vi "MattFileCreator-v9.vi"(6 "Comments":T5, 8 "Input Array":dbl[](array[numeric]), 9 "File path":path, 10 "table":string, 11 "connection reference":T6) -> (0 "error out":errorcluster, 3 "connection reference out":T6)   [LabVIEW 2014]
uses:
  <vilib>/addons/database/Connection.llb/Conn ObjectReference.ctl
  <vilib>/addons/database/NI_Database_API.lvlib
panel:
  out "output cluster 4":T1
  out "output cluster 3":T2
  out "output cluster 2":T3
  out "output cluster":T4
  in  "Database input":T7
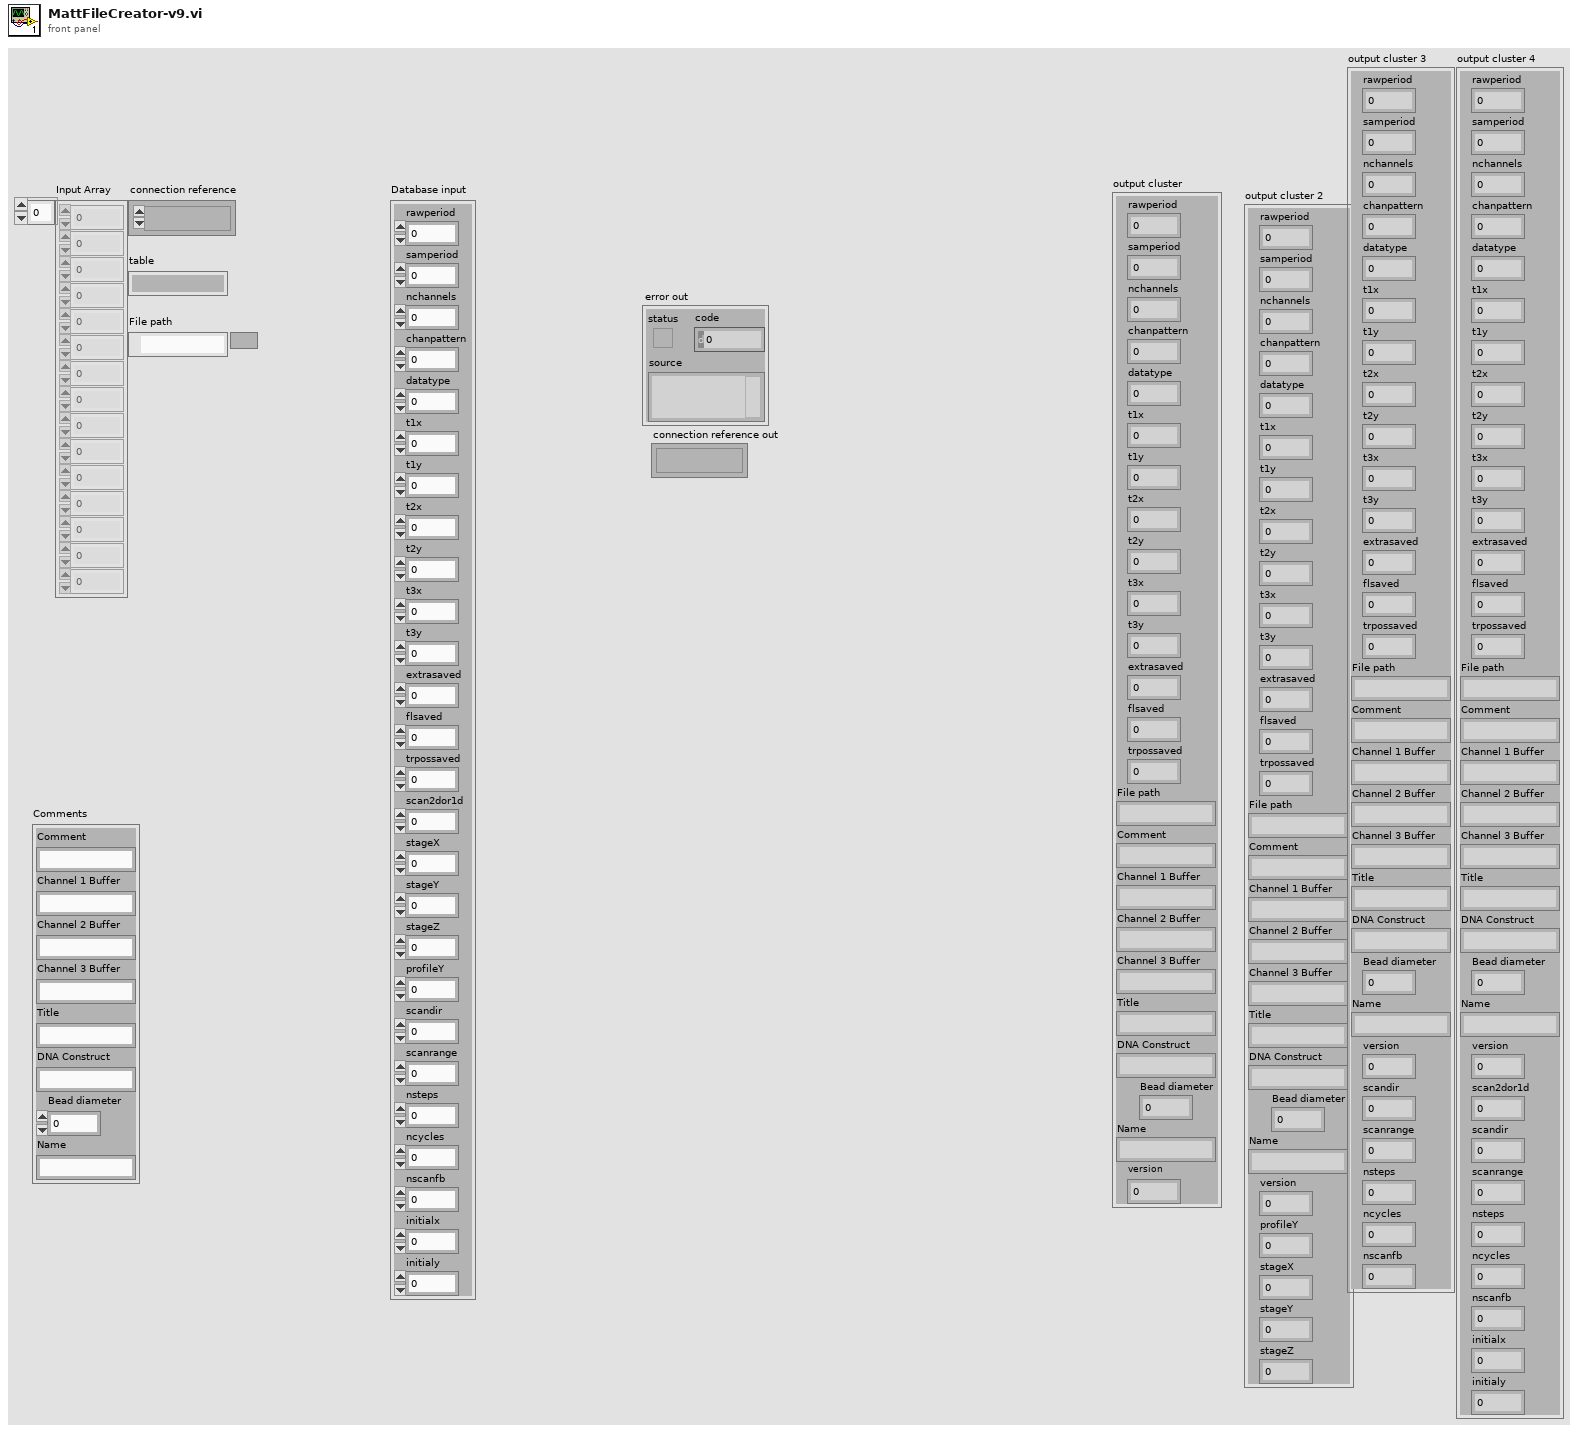
[diagram p1: front panel]
types:
  T1 = cluster{"rawperiod":dbl, "samperiod":dbl, "nchannels":dbl, "chanpattern":dbl, "datatype":dbl, "t1x":dbl, "t1y":dbl, "t2x":dbl, "t2y":dbl, "t3x":dbl, "t3y":dbl, "extrasaved":dbl, "flsaved":dbl, "trpossaved":dbl, "File path":string, "Comment":string, "Channel 1 Buffer":string, "Channel 2 Buffer":string, "Channel 3 Buffer":string, "Title":string, "DNA Construct":string, "Bead diameter":dbl, "Name":string, "version":i32, "scan2dor1d":dbl, "scandir":dbl, "scanrange":dbl, "nsteps":dbl, "ncycles":dbl, "nscanfb":dbl, "initialx":dbl, "initialy":dbl}
  T2 = cluster{"rawperiod":dbl, "samperiod":dbl, "nchannels":dbl, "chanpattern":dbl, "datatype":dbl, "t1x":dbl, "t1y":dbl, "t2x":dbl, "t2y":dbl, "t3x":dbl, "t3y":dbl, "extrasaved":dbl, "flsaved":dbl, "trpossaved":dbl, "File path":string, "Comment":string, "Channel 1 Buffer":string, "Channel 2 Buffer":string, "Channel 3 Buffer":string, "Title":string, "DNA Construct":string, "Bead diameter":dbl, "Name":string, "version":i32, "scandir":dbl, "scanrange":dbl, "nsteps":dbl, "ncycles":dbl, "nscanfb":dbl}
  T3 = cluster{"rawperiod":dbl, "samperiod":dbl, "nchannels":dbl, "chanpattern":dbl, "datatype":dbl, "t1x":dbl, "t1y":dbl, "t2x":dbl, "t2y":dbl, "t3x":dbl, "t3y":dbl, "extrasaved":dbl, "flsaved":dbl, "trpossaved":dbl, "File path":string, "Comment":string, "Channel 1 Buffer":string, "Channel 2 Buffer":string, "Channel 3 Buffer":string, "Title":string, "DNA Construct":string, "Bead diameter":dbl, "Name":string, "version":i32, "profileY":dbl, "stageX":dbl, "stageY":dbl, "stageZ":dbl}
  T4 = cluster{"rawperiod":dbl, "samperiod":dbl, "nchannels":dbl, "chanpattern":dbl, "datatype":dbl, "t1x":dbl, "t1y":dbl, "t2x":dbl, "t2y":dbl, "t3x":dbl, "t3y":dbl, "extrasaved":dbl, "flsaved":dbl, "trpossaved":dbl, "File path":string, "Comment":string, "Channel 1 Buffer":string, "Channel 2 Buffer":string, "Channel 3 Buffer":string, "Title":string, "DNA Construct":string, "Bead diameter":dbl, "Name":string, "version":i32}
  T5 = cluster{"Comment":string, "Channel 1 Buffer":string, "Channel 2 Buffer":string, "Channel 3 Buffer":string, "Title":string, "DNA Construct":string, "Bead diameter":dbl, "Name":string}
  T6 = typedef "NI_Database_API.lvlib/Conn ObjectReference.ctl" = refnum<k1>
  T7 = cluster{"rawperiod":dbl, "samperiod":dbl, "nchannels":dbl, "chanpattern":dbl, "datatype":dbl, "t1x":dbl, "t1y":dbl, "t2x":dbl, "t2y":dbl, "t3x":dbl, "t3y":dbl, "extrasaved":dbl, "flsaved":dbl, "trpossaved":dbl, "scan2dor1d":dbl, "stageX":dbl, "stageY":dbl, "stageZ":dbl, "profileY":dbl, "scandir":dbl, "scanrange":dbl, "nsteps":dbl, "ncycles":dbl, "nscanfb":dbl, "initialx":dbl, "initialy":dbl}
  T8 = cluster{"Input Array[0]":dbl, "Input Array[1]":dbl, "Input Array[2]":dbl, "Input Array[3]":dbl, "Input Array[4]":dbl, "Input Array[5]":dbl, "Input Array[6]":dbl, "Input Array[7]":dbl, "Input Array[8]":dbl, "Input Array[9]":dbl, "Input Array[10]":dbl, "Input Array[11]":dbl, "Input Array[12]":dbl, "Input Array[13]":dbl, "Input Array[14]":dbl, "Input Array[15]":dbl, "Input Array[16]":dbl, "Input Array[17]":dbl, "Input Array[18]":dbl, "Input Array[19]":dbl}
  T9 = cluster{"rawperiod":dbl, "samperiod":dbl, "nchannels":dbl, "chanpattern":dbl, "datatype":dbl, "t1x":dbl, "t1y":dbl, "t2x":dbl, "t2y":dbl, "t3x":dbl, "t3y":dbl, "extrasaved":dbl, "flsaved":dbl, "trpossaved":dbl, string, "Comment":string, "Channel 1 Buffer":string, "Channel 2 Buffer":string, "Channel 3 Buffer":string, "Title":string, "DNA Construct":string, "Bead diameter":dbl, "Name":string, "version":i32}
  T10 = cluster{"rawperiod":dbl, "samperiod":dbl, "nchannels":dbl, "chanpattern":dbl, "datatype":dbl, "t1x":dbl, "t1y":dbl, "t2x":dbl, "t2y":dbl, "t3x":dbl, "t3y":dbl, "extrasaved":dbl, "flsaved":dbl, "trpossaved":dbl, string, "Comment":string, "Channel 1 Buffer":string, "Channel 2 Buffer":string, "Channel 3 Buffer":string, "Title":string, "DNA Construct":string, "Bead diameter":dbl, "Name":string, "version":i32, "profileY":dbl, "stageX":dbl, "stageY":dbl, "stageZ":dbl}
  T11 = cluster{"Input Array[0]":dbl, "Input Array[1]":dbl, "Input Array[2]":dbl, "Input Array[3]":dbl, "Input Array[4]":dbl, "Input Array[5]":dbl, "Input Array[6]":dbl, "Input Array[7]":dbl, "Input Array[8]":dbl, "Input Array[9]":dbl, "Input Array[10]":dbl, "Input Array[11]":dbl, "Input Array[12]":dbl, "Input Array[13]":dbl, "Input Array[14]":dbl, "Input Array[15]":dbl, "Input Array[16]":dbl, "Input Array[17]":dbl, "Input Array[18]":dbl, "Input Array[19]":dbl, "Input Array[20]":dbl, "Input Array[21]":dbl, "Input Array[22]":dbl, "Input Array[23]":dbl, "Input Array[24]":dbl}
  T12 = cluster{"rawperiod":dbl, "samperiod":dbl, "nchannels":dbl, "chanpattern":dbl, "datatype":dbl, "t1x":dbl, "t1y":dbl, "t2x":dbl, "t2y":dbl, "t3x":dbl, "t3y":dbl, "extrasaved":dbl, "flsaved":dbl, "trpossaved":dbl, string, "Comment":string, "Channel 1 Buffer":string, "Channel 2 Buffer":string, "Channel 3 Buffer":string, "Title":string, "DNA Construct":string, "Bead diameter":dbl, "Name":string, "version":i32, "scandir":dbl, "scanrange":dbl, "nsteps":dbl, "ncycles":dbl, "nscanfb":dbl}
  T13 = cluster{"rawperiod":dbl, "samperiod":dbl, "nchannels":dbl, "chanpattern":dbl, "datatype":dbl, "t1x":dbl, "t1y":dbl, "t2x":dbl, "t2y":dbl, "t3x":dbl, "t3y":dbl, "extrasaved":dbl, "flsaved":dbl, "trpossaved":dbl, string, "Comment":string, "Channel 1 Buffer":string, "Channel 2 Buffer":string, "Channel 3 Buffer":string, "Title":string, "DNA Construct":string, "Bead diameter":dbl, "Name":string, "version":i32, "scan2dor1d":dbl, "scandir":dbl, "scanrange":dbl, "nsteps":dbl, "ncycles":dbl, "nscanfb":dbl, "initialx":dbl, "initialy":dbl}
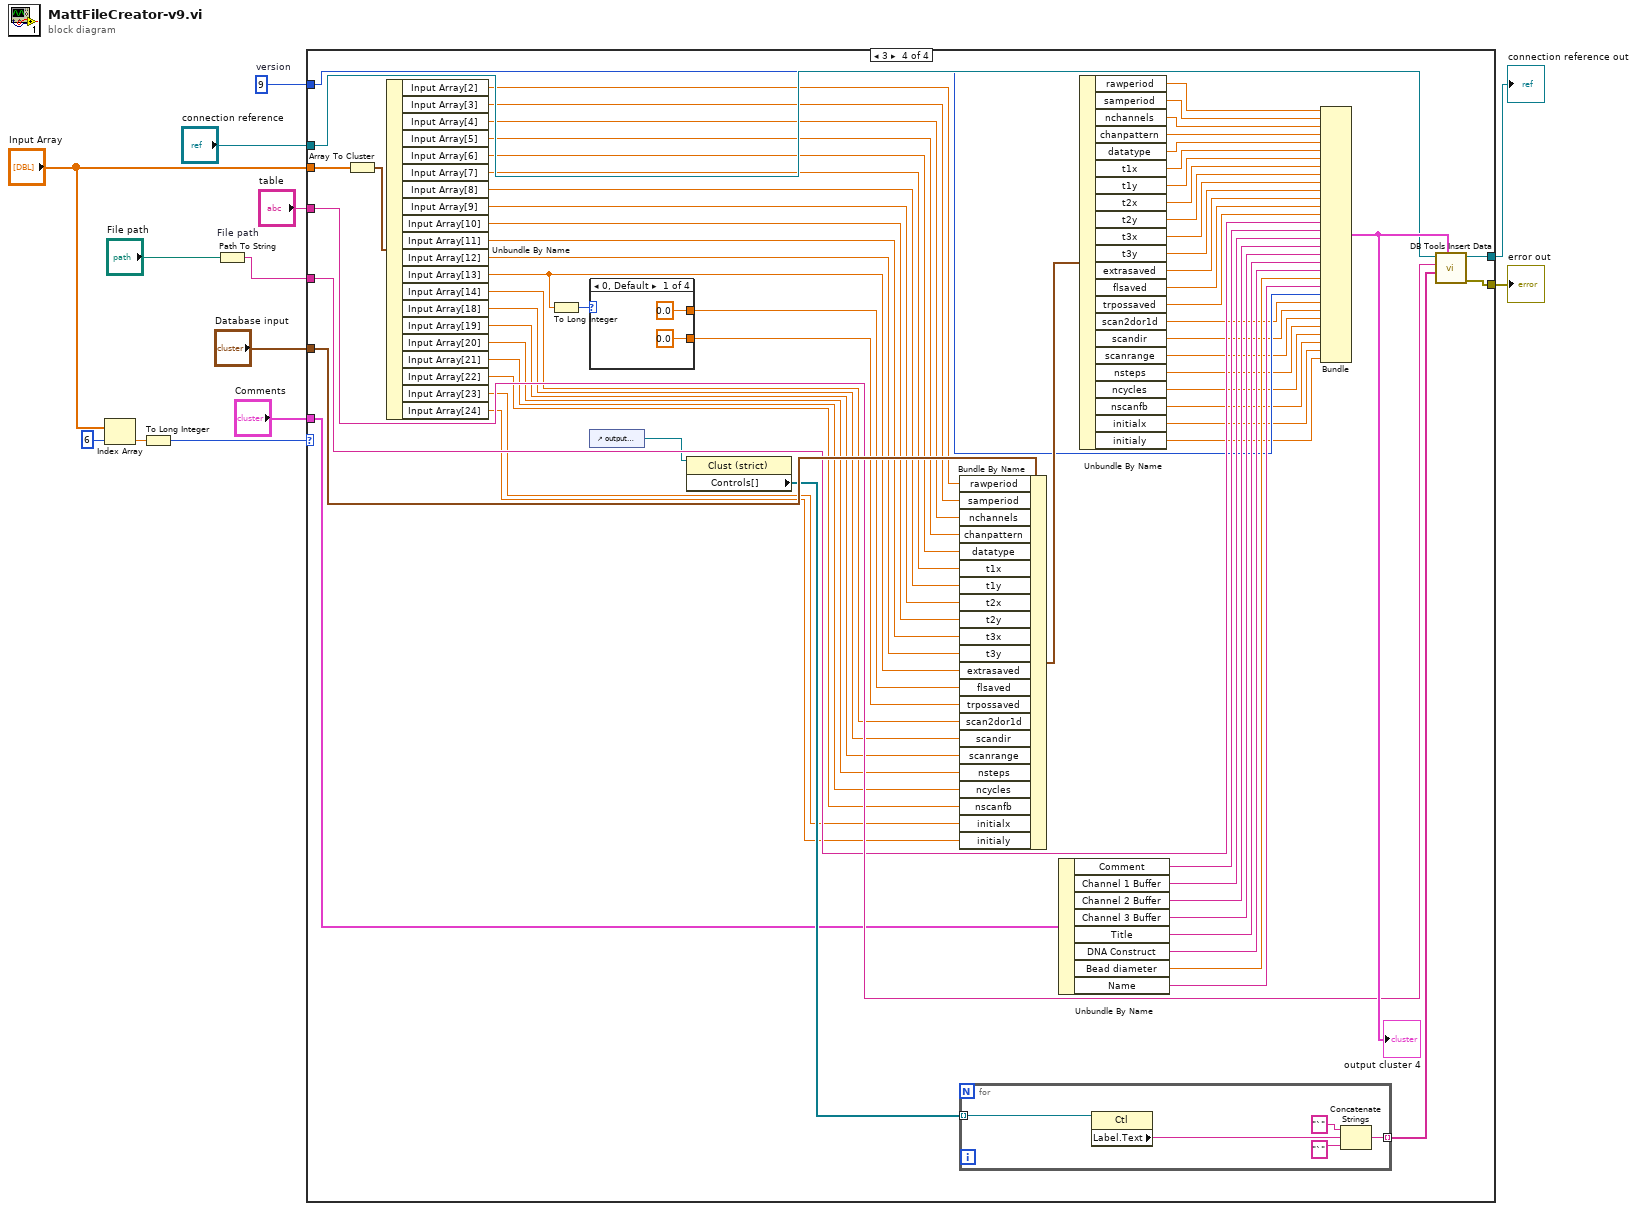
[diagram p0: block diagram]
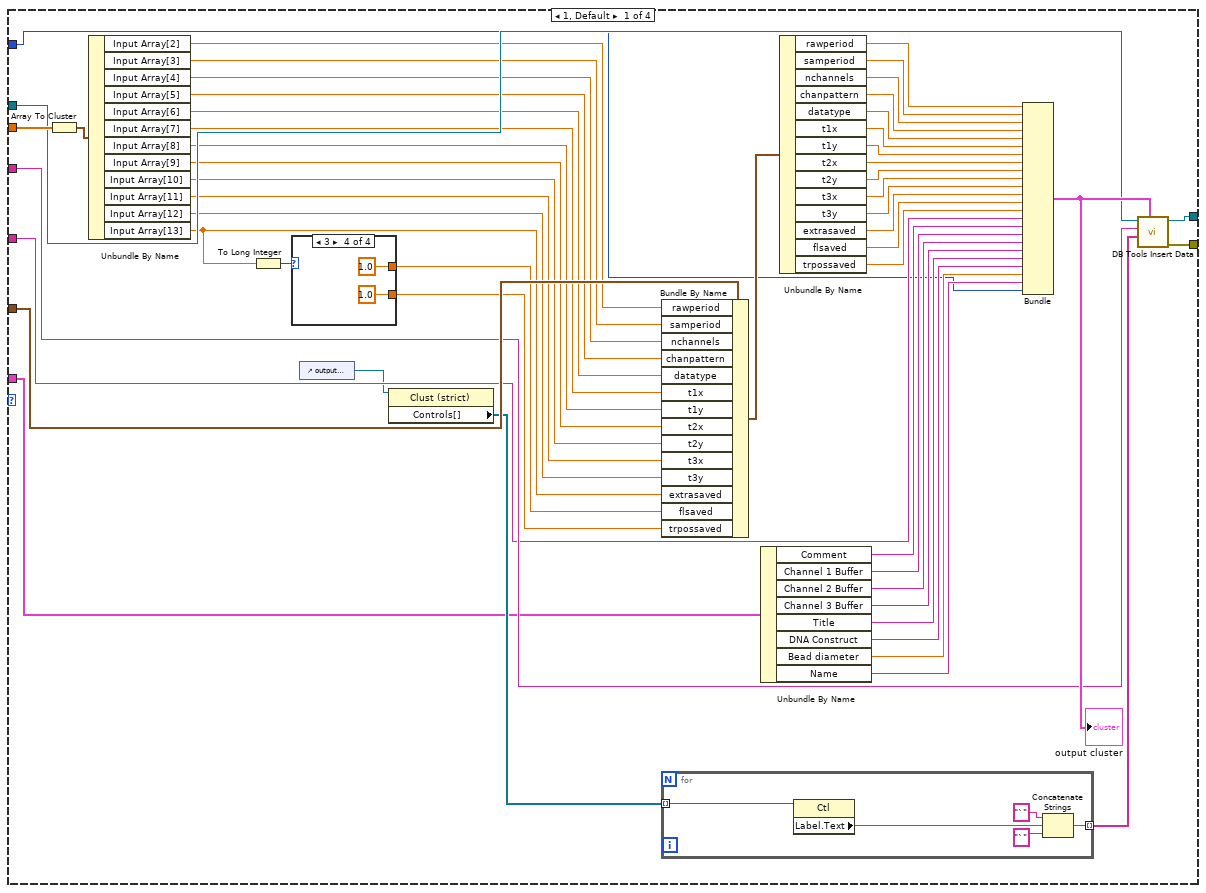
[diagram p2: hidden frame]
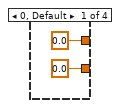
[diagram p3: hidden frame]
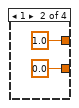
[diagram p4: hidden frame]
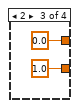
[diagram p5: hidden frame]
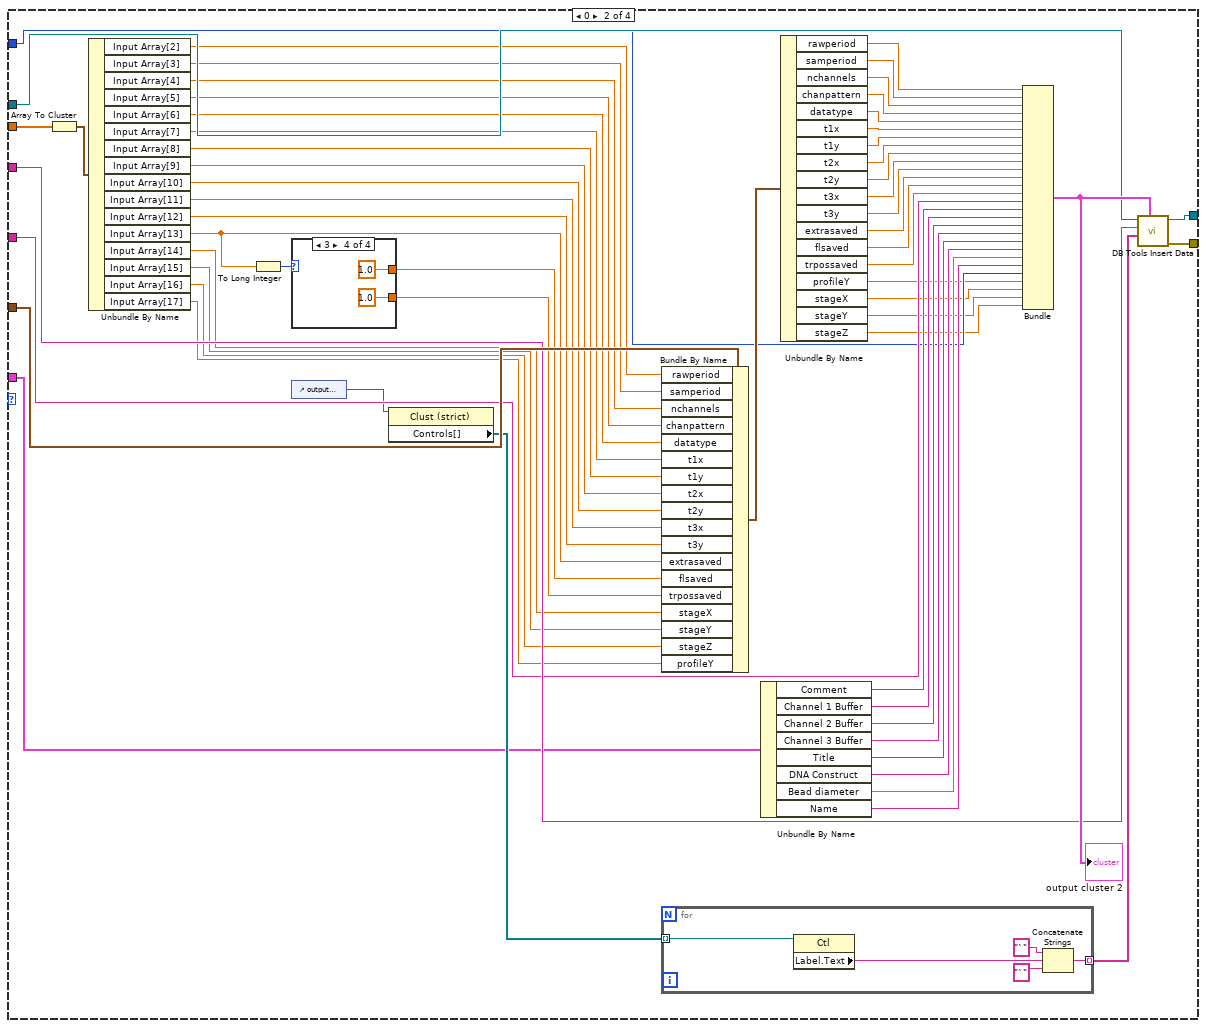
[diagram p6: hidden frame]
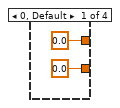
[diagram p7: hidden frame]
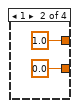
[diagram p8: hidden frame]
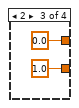
[diagram p9: hidden frame]
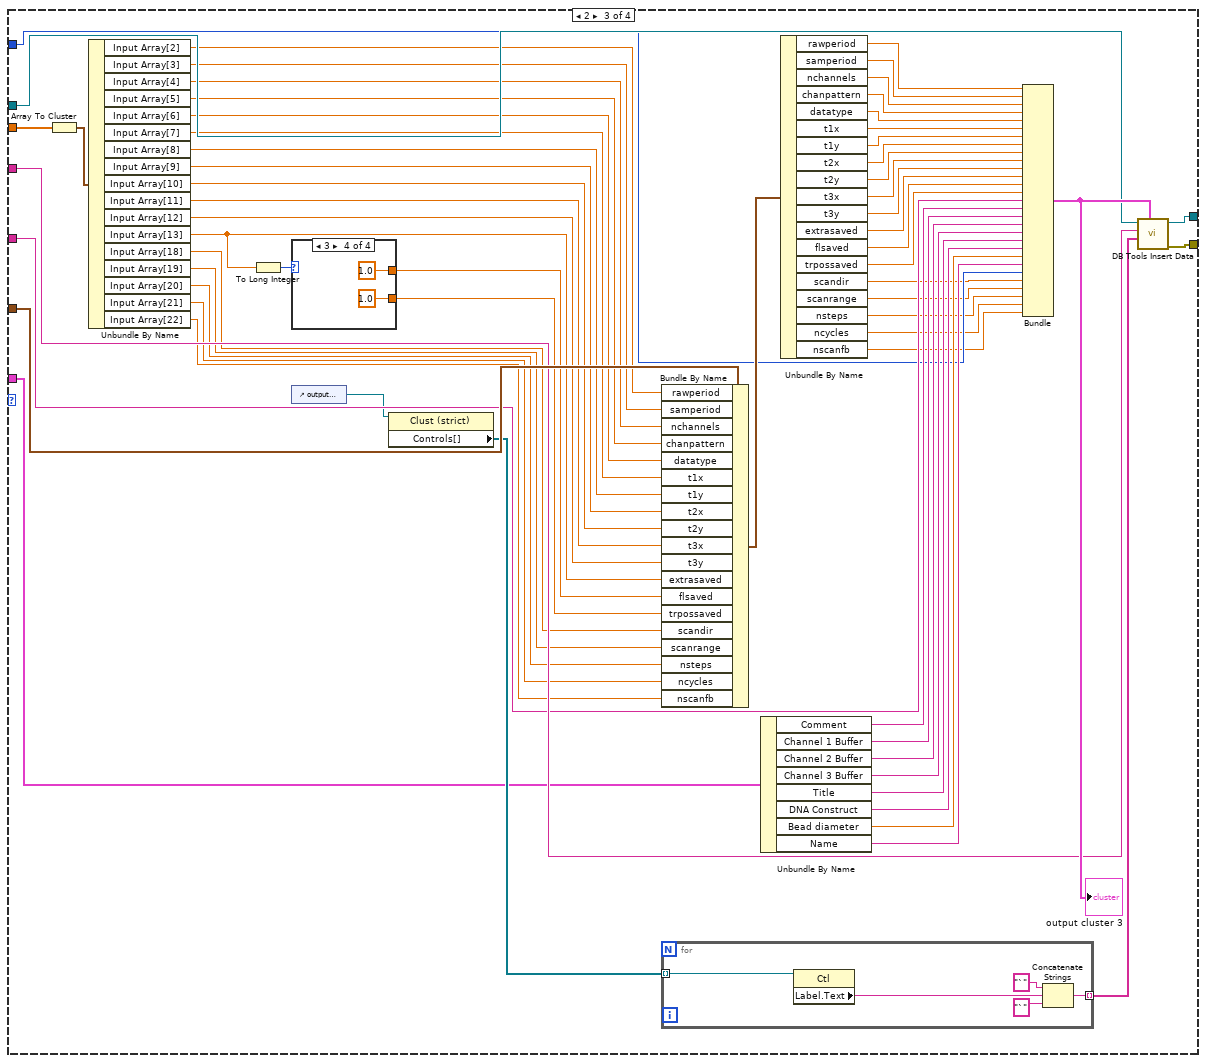
[diagram p10: hidden frame]
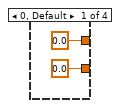
[diagram p11: hidden frame]
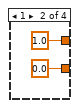
[diagram p12: hidden frame]
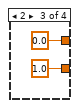
[diagram p13: hidden frame]
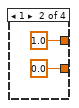
[diagram p14: hidden frame]
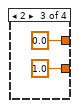
[diagram p15: hidden frame]
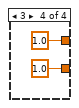
[diagram p16: hidden frame]
diagram:
  w3 = 9  # version
  n1 = Index Array(array="Input Array", index=6) -> (element=w12:dbl)
  n2 = To Long Integer(number=w12) -> (32bit integer=w11:i32)
  n3 = Path To String "File path"(path="File path") -> (string=w1:string)
  n4 = case shown="3" w11 {
    tunnel: "Database input" -> [w65 w138 w213 w294]
    tunnel: "Input Array" -> [w64 w137 w212 w293]
    tunnel: "connection reference" -> [w44 w117 w192 w273]
    tunnel: "table" -> [w43 w116 w191 w272]
    tunnel: [w42 w115 w190 w271] -> w6
    tunnel: [w41 w114 w189 w270] -> w5
    tunnel: w1 -> [w40 w113 w188 w269]
    tunnel: "Comments" -> [w39 w112 w187 w268]
    tunnel: w3 -> [w30 w103 w178 w259]
    frame 1, Default {
      n5 = Array To Cluster(array=w64) -> (cluster=w63:T8)
      n6 = Unbundle By Name(w63) -> ("Input Array[2]"=w28:dbl, "Input Array[3]"=w27:dbl, "Input Array[4]"=w26:dbl, "Input Array[5]"=w25:dbl, "Input Array[6]"=w24:dbl, "Input Array[7]"=w23:dbl, "Input Array[8]"=w22:dbl, "Input Array[9]"=w21:dbl, "Input Array[10]"=w20:dbl, "Input Array[11]"=w19:dbl, "Input Array[12]"=w18:dbl, "Input Array[13]"=w16:dbl)
      n7 = To Long Integer(number=w16) -> (32bit integer=w17:i32)
      n8 = case shown="3" w17 {
        tunnel: [0.0 1.0 0.0 1.0] -> w15
        tunnel: [0.0 0.0 1.0 1.0] -> w14
        frame 0, Default {
        }
        frame 1 {
        }
        frame 2 {
        }
        frame 3 {
        }
      }
      n9 = control-ref of="output cluster"() -> (w29:refnum<vi>)
      n10 = property class="Clust (strict)"(reference=w29) -> ("Controls[]"=w47:refnum<vi>[])  [unwired: 1 in, 2 out]
      n11 = Bundle By Name(cluster=w65, "rawperiod"=w28, "samperiod"=w27, "nchannels"=w26, "chanpattern"=w25, "datatype"=w24, "t1x"=w23, "t1y"=w22, "t2x"=w21, "t2y"=w20, "t3x"=w19, "t3y"=w18, "extrasaved"=w16, "flsaved"=w15, "trpossaved"=w14) -> (w62:T7)
      n12 = for {
        tunnel: w47 -> [w78] mode=indexing
        tunnel: [w74] -> w46 mode=indexing
        n13 = property class="Ctl"(reference=w78) -> ("Label.Text"=w77:string)  [unwired: 1 in, 2 out]
        n14 = Concatenate Strings("`" ("string"), w77, "`" ("string")) -> (w74:string)
      }
      n15 = Unbundle By Name(w39) -> ("Comment"=w38:string, "Channel 1 Buffer"=w37:string, "Channel 2 Buffer"=w36:string, "Channel 3 Buffer"=w35:string, "Title"=w34:string, "DNA Construct"=w33:string, "Bead diameter"=w32:dbl, "Name"=w31:string)
      n16 = Unbundle By Name(w62) -> ("rawperiod"=w61:dbl, "samperiod"=w60:dbl, "nchannels"=w59:dbl, "chanpattern"=w58:dbl, "datatype"=w57:dbl, "t1x"=w56:dbl, "t1y"=w55:dbl, "t2x"=w54:dbl, "t2y"=w53:dbl, "t3x"=w52:dbl, "t3y"=w51:dbl, "extrasaved"=w50:dbl, "flsaved"=w49:dbl, "trpossaved"=w48:dbl)
      n17 = Bundle("rawperiod"=w61, "samperiod"=w60, "nchannels"=w59, "chanpattern"=w58, "datatype"=w57, "t1x"=w56, "t1y"=w55, "t2x"=w54, "t2y"=w53, "t3x"=w52, "t3y"=w51, "extrasaved"=w50, "flsaved"=w49, "trpossaved"=w48, w40, "Comment"=w38, "Channel 1 Buffer"=w37, "Channel 2 Buffer"=w36, "Channel 3 Buffer"=w35, "Title"=w34, "DNA Construct"=w33, "Bead diameter"=w32, "Name"=w31, "version"=w30) -> (w45:T9)  [unwired: 1 in]
      "output cluster" <- w45
      n18 = call <vilib>:"DB Tools Insert Data.vi"("data"=w45, "columns"=w46, "table"=w43, "connection reference"=w44) -> ("error out"=w42:errorcluster, "connection reference out"=w41:T6)  [unwired: 6 in]
    }
    frame 0 {
      n19 = Array To Cluster(array=w137) -> (cluster=w136:T8)
      n20 = Unbundle By Name(w136) -> ("Input Array[2]"=w102:dbl, "Input Array[3]"=w101:dbl, "Input Array[4]"=w100:dbl, "Input Array[5]"=w99:dbl, "Input Array[6]"=w98:dbl, "Input Array[7]"=w97:dbl, "Input Array[8]"=w96:dbl, "Input Array[9]"=w95:dbl, "Input Array[10]"=w94:dbl, "Input Array[11]"=w93:dbl, "Input Array[12]"=w92:dbl, "Input Array[13]"=w90:dbl, "Input Array[14]"=w87:dbl, "Input Array[15]"=w86:dbl, "Input Array[16]"=w85:dbl, "Input Array[17]"=w84:dbl)
      n21 = To Long Integer(number=w90) -> (32bit integer=w91:i32)
      n22 = case shown="3" w91 {
        tunnel: [0.0 1.0 0.0 1.0] -> w89
        tunnel: [0.0 0.0 1.0 1.0] -> w88
        frame 0, Default {
        }
        frame 1 {
        }
        frame 2 {
        }
        frame 3 {
        }
      }
      n23 = control-ref of="output cluster 2"() -> (w79:refnum<vi>)
      n24 = property class="Clust (strict)"(reference=w79) -> ("Controls[]"=w120:refnum<vi>[])  [unwired: 1 in, 2 out]
      n25 = Bundle By Name(cluster=w138, "rawperiod"=w102, "samperiod"=w101, "nchannels"=w100, "chanpattern"=w99, "datatype"=w98, "t1x"=w97, "t1y"=w96, "t2x"=w95, "t2y"=w94, "t3x"=w93, "t3y"=w92, "extrasaved"=w90, "flsaved"=w89, "trpossaved"=w88, "stageX"=w87, "stageY"=w86, "stageZ"=w85, "profileY"=w84) -> (w135:T7)
      n26 = for {
        tunnel: w120 -> [w151] mode=indexing
        tunnel: [w147] -> w119 mode=indexing
        n27 = property class="Ctl"(reference=w151) -> ("Label.Text"=w150:string)  [unwired: 1 in, 2 out]
        n28 = Concatenate Strings("`" ("string"), w150, "`" ("string")) -> (w147:string)
      }
      n29 = Unbundle By Name(w112) -> ("Comment"=w111:string, "Channel 1 Buffer"=w110:string, "Channel 2 Buffer"=w109:string, "Channel 3 Buffer"=w108:string, "Title"=w107:string, "DNA Construct"=w106:string, "Bead diameter"=w105:dbl, "Name"=w104:string)
      n30 = Unbundle By Name(w135) -> ("rawperiod"=w134:dbl, "samperiod"=w133:dbl, "nchannels"=w132:dbl, "chanpattern"=w131:dbl, "datatype"=w130:dbl, "t1x"=w129:dbl, "t1y"=w128:dbl, "t2x"=w127:dbl, "t2y"=w126:dbl, "t3x"=w125:dbl, "t3y"=w124:dbl, "extrasaved"=w123:dbl, "flsaved"=w122:dbl, "trpossaved"=w121:dbl, "profileY"=w83:dbl, "stageX"=w82:dbl, "stageY"=w81:dbl, "stageZ"=w80:dbl)
      n31 = Bundle("rawperiod"=w134, "samperiod"=w133, "nchannels"=w132, "chanpattern"=w131, "datatype"=w130, "t1x"=w129, "t1y"=w128, "t2x"=w127, "t2y"=w126, "t3x"=w125, "t3y"=w124, "extrasaved"=w123, "flsaved"=w122, "trpossaved"=w121, w113, "Comment"=w111, "Channel 1 Buffer"=w110, "Channel 2 Buffer"=w109, "Channel 3 Buffer"=w108, "Title"=w107, "DNA Construct"=w106, "Bead diameter"=w105, "Name"=w104, "version"=w103, "profileY"=w83, "stageX"=w82, "stageY"=w81, "stageZ"=w80) -> (w118:T10)  [unwired: 1 in]
      "output cluster 2" <- w118
      n32 = call <vilib>:"DB Tools Insert Data.vi"("data"=w118, "columns"=w119, "table"=w116, "connection reference"=w117) -> ("error out"=w115:errorcluster, "connection reference out"=w114:T6)  [unwired: 6 in]
    }
    frame 2 {
      n33 = Array To Cluster(array=w212) -> (cluster=w211:T11)
      n34 = Unbundle By Name(w211) -> ("Input Array[2]"=w177:dbl, "Input Array[3]"=w176:dbl, "Input Array[4]"=w175:dbl, "Input Array[5]"=w174:dbl, "Input Array[6]"=w173:dbl, "Input Array[7]"=w172:dbl, "Input Array[8]"=w171:dbl, "Input Array[9]"=w170:dbl, "Input Array[10]"=w169:dbl, "Input Array[11]"=w168:dbl, "Input Array[12]"=w167:dbl, "Input Array[13]"=w165:dbl, "Input Array[18]"=w162:dbl, "Input Array[19]"=w161:dbl, "Input Array[20]"=w160:dbl, "Input Array[21]"=w159:dbl, "Input Array[22]"=w158:dbl)
      n35 = To Long Integer(number=w165) -> (32bit integer=w166:i32)
      n36 = case shown="3" w166 {
        tunnel: [0.0 1.0 0.0 1.0] -> w164
        tunnel: [0.0 0.0 1.0 1.0] -> w163
        frame 0, Default {
        }
        frame 1 {
        }
        frame 2 {
        }
        frame 3 {
        }
      }
      n37 = control-ref of="output cluster 3"() -> (w152:refnum<vi>)
      n38 = property class="Clust (strict)"(reference=w152) -> ("Controls[]"=w195:refnum<vi>[])  [unwired: 1 in, 2 out]
      n39 = Bundle By Name(cluster=w213, "rawperiod"=w177, "samperiod"=w176, "nchannels"=w175, "chanpattern"=w174, "datatype"=w173, "t1x"=w172, "t1y"=w171, "t2x"=w170, "t2y"=w169, "t3x"=w168, "t3y"=w167, "extrasaved"=w165, "flsaved"=w164, "trpossaved"=w163, "scandir"=w162, "scanrange"=w161, "nsteps"=w160, "ncycles"=w159, "nscanfb"=w158) -> (w210:T7)
      n40 = for {
        tunnel: w195 -> [w226] mode=indexing
        tunnel: [w222] -> w194 mode=indexing
        n41 = property class="Ctl"(reference=w226) -> ("Label.Text"=w225:string)  [unwired: 1 in, 2 out]
        n42 = Concatenate Strings("`" ("string"), w225, "`" ("string")) -> (w222:string)
      }
      n43 = Unbundle By Name(w187) -> ("Comment"=w186:string, "Channel 1 Buffer"=w185:string, "Channel 2 Buffer"=w184:string, "Channel 3 Buffer"=w183:string, "Title"=w182:string, "DNA Construct"=w181:string, "Bead diameter"=w180:dbl, "Name"=w179:string)
      n44 = Unbundle By Name(w210) -> ("rawperiod"=w209:dbl, "samperiod"=w208:dbl, "nchannels"=w207:dbl, "chanpattern"=w206:dbl, "datatype"=w205:dbl, "t1x"=w204:dbl, "t1y"=w203:dbl, "t2x"=w202:dbl, "t2y"=w201:dbl, "t3x"=w200:dbl, "t3y"=w199:dbl, "extrasaved"=w198:dbl, "flsaved"=w197:dbl, "trpossaved"=w196:dbl, "scandir"=w157:dbl, "scanrange"=w156:dbl, "nsteps"=w155:dbl, "ncycles"=w154:dbl, "nscanfb"=w153:dbl)
      n45 = Bundle("rawperiod"=w209, "samperiod"=w208, "nchannels"=w207, "chanpattern"=w206, "datatype"=w205, "t1x"=w204, "t1y"=w203, "t2x"=w202, "t2y"=w201, "t3x"=w200, "t3y"=w199, "extrasaved"=w198, "flsaved"=w197, "trpossaved"=w196, w188, "Comment"=w186, "Channel 1 Buffer"=w185, "Channel 2 Buffer"=w184, "Channel 3 Buffer"=w183, "Title"=w182, "DNA Construct"=w181, "Bead diameter"=w180, "Name"=w179, "version"=w178, "scandir"=w157, "scanrange"=w156, "nsteps"=w155, "ncycles"=w154, "nscanfb"=w153) -> (w193:T12)  [unwired: 1 in]
      "output cluster 3" <- w193
      n46 = call <vilib>:"DB Tools Insert Data.vi"("data"=w193, "columns"=w194, "table"=w191, "connection reference"=w192) -> ("error out"=w190:errorcluster, "connection reference out"=w189:T6)  [unwired: 6 in]
    }
    frame 3 {
      n47 = Array To Cluster(array=w293) -> (cluster=w292:T11)
      n48 = Unbundle By Name(w292) -> ("Input Array[2]"=w258:dbl, "Input Array[3]"=w257:dbl, "Input Array[4]"=w256:dbl, "Input Array[5]"=w255:dbl, "Input Array[6]"=w254:dbl, "Input Array[7]"=w253:dbl, "Input Array[8]"=w252:dbl, "Input Array[9]"=w251:dbl, "Input Array[10]"=w250:dbl, "Input Array[11]"=w249:dbl, "Input Array[12]"=w248:dbl, "Input Array[13]"=w246:dbl, "Input Array[14]"=w235:dbl, "Input Array[18]"=w234:dbl, "Input Array[19]"=w233:dbl, "Input Array[20]"=w232:dbl, "Input Array[21]"=w231:dbl, "Input Array[22]"=w230:dbl, "Input Array[23]"=w229:dbl, "Input Array[24]"=w228:dbl)
      n49 = To Long Integer(number=w246) -> (32bit integer=w247:i32)
      n50 = case shown="0, Default" w247 {
        tunnel: [0.0 1.0 0.0 1.0] -> w245
        tunnel: [0.0 0.0 1.0 1.0] -> w244
        frame 0, Default {
        }
        frame 1 {
        }
        frame 2 {
        }
        frame 3 {
        }
      }
      n51 = control-ref of="output cluster 4"() -> (w227:refnum<vi>)
      n52 = property class="Clust (strict)"(reference=w227) -> ("Controls[]"=w276:refnum<vi>[])  [unwired: 1 in, 2 out]
      n53 = Bundle By Name(cluster=w294, "rawperiod"=w258, "samperiod"=w257, "nchannels"=w256, "chanpattern"=w255, "datatype"=w254, "t1x"=w253, "t1y"=w252, "t2x"=w251, "t2y"=w250, "t3x"=w249, "t3y"=w248, "extrasaved"=w246, "flsaved"=w245, "trpossaved"=w244, "scan2dor1d"=w235, "scandir"=w234, "scanrange"=w233, "nsteps"=w232, "ncycles"=w231, "nscanfb"=w230, "initialx"=w229, "initialy"=w228) -> (w291:T7)
      n54 = for {
        tunnel: w276 -> [w307] mode=indexing
        tunnel: [w303] -> w275 mode=indexing
        n55 = property class="Ctl"(reference=w307) -> ("Label.Text"=w306:string)  [unwired: 1 in, 2 out]
        n56 = Concatenate Strings("`" ("string"), w306, "`" ("string")) -> (w303:string)
      }
      n57 = Unbundle By Name(w268) -> ("Comment"=w267:string, "Channel 1 Buffer"=w266:string, "Channel 2 Buffer"=w265:string, "Channel 3 Buffer"=w264:string, "Title"=w263:string, "DNA Construct"=w262:string, "Bead diameter"=w261:dbl, "Name"=w260:string)
      n58 = Unbundle By Name(w291) -> ("rawperiod"=w290:dbl, "samperiod"=w289:dbl, "nchannels"=w288:dbl, "chanpattern"=w287:dbl, "datatype"=w286:dbl, "t1x"=w285:dbl, "t1y"=w284:dbl, "t2x"=w283:dbl, "t2y"=w282:dbl, "t3x"=w281:dbl, "t3y"=w280:dbl, "extrasaved"=w279:dbl, "flsaved"=w278:dbl, "trpossaved"=w277:dbl, "scan2dor1d"=w243:dbl, "scandir"=w242:dbl, "scanrange"=w241:dbl, "nsteps"=w240:dbl, "ncycles"=w239:dbl, "nscanfb"=w238:dbl, "initialx"=w237:dbl, "initialy"=w236:dbl)
      n59 = Bundle("rawperiod"=w290, "samperiod"=w289, "nchannels"=w288, "chanpattern"=w287, "datatype"=w286, "t1x"=w285, "t1y"=w284, "t2x"=w283, "t2y"=w282, "t3x"=w281, "t3y"=w280, "extrasaved"=w279, "flsaved"=w278, "trpossaved"=w277, w269, "Comment"=w267, "Channel 1 Buffer"=w266, "Channel 2 Buffer"=w265, "Channel 3 Buffer"=w264, "Title"=w263, "DNA Construct"=w262, "Bead diameter"=w261, "Name"=w260, "version"=w259, "scan2dor1d"=w243, "scandir"=w242, "scanrange"=w241, "nsteps"=w240, "ncycles"=w239, "nscanfb"=w238, "initialx"=w237, "initialy"=w236) -> (w274:T13)  [unwired: 1 in]
      "output cluster 4" <- w274
      n60 = call <vilib>:"DB Tools Insert Data.vi"("data"=w274, "columns"=w275, "table"=w272, "connection reference"=w273) -> ("error out"=w271:errorcluster, "connection reference out"=w270:T6)  [unwired: 6 in]
    }
  }
  "error out" <- w6
  "connection reference out" <- w5
